vi "Init.vi"(8 "error in (no error)":errorcluster, 9 "C4209 Cfg":T1={"ResourceName"="", "Enable"=FALSE, "Channel"=1, "CalFileName"="", "MeasName"="", "TempDatFile"="", "Power, dBm"=-30.0, "NumPoints"=201, "Start Freq, Hz"=5000000000.0, "Stop Freq, Hz"=6000000000.0, "NumAverages"=20, "Sweep Type"=0} {"Sweep Type" items=["Linear Frequency", "Log Frequency", "Power Sweep", "CW Time"]; "Stop Freq, Hz" format="%_3p"; "Start Freq, Hz" format="%_3p"}, 11 "C4209 PNA":refnum<class "C4209 PNA.lvclass">) -> (0 "error out":errorcluster, 3 "C4209 PNA out":refnum<class "C4209 PNA.lvclass">)   [LabVIEW 2017, in "C4209 PNA.lvclass"]
uses:
  C4209 PNA.lvclass
  N5222A PNA/N5222AConfig.ctl
  C4209 PNA.lvclass/C4209 PNA.ctl
  <instrlib>/CMT S2 Series VNA/CMT S2 Series VNA.lvlib
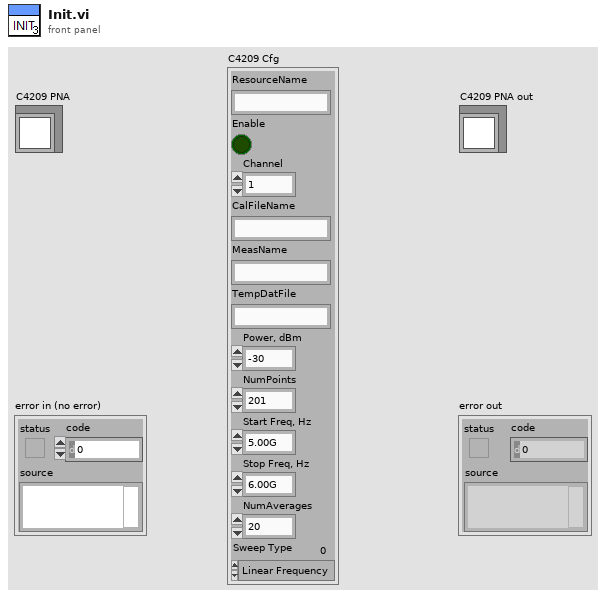
[diagram p1: front panel]
types:
  T1 = typedef "N5222AConfig.ctl" = cluster{"ResourceName":string, "Enable":bool, "Channel":i32, "CalFileName":string, "MeasName":string, "TempDatFile":string, "Power, dBm":dbl, "NumPoints":i32, "Start Freq, Hz":dbl, "Stop Freq, Hz":dbl, "NumAverages":i32, "Sweep Type":i32}
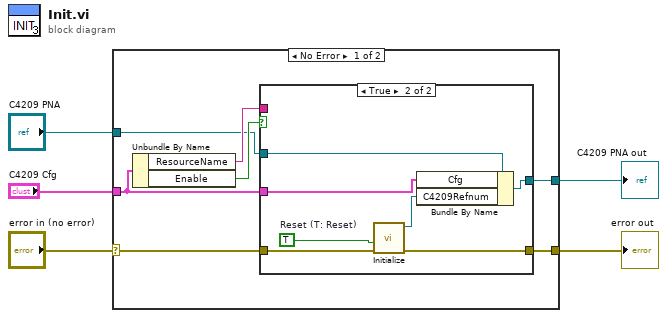
[diagram p0: block diagram]
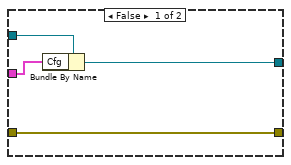
[diagram p2: hidden frame]
diagram:
  n1 = case shown="No Error" "error in (no error)" {
    selector: "error in (no error)" -> [w7 w25]
    tunnel: [w8 w25] -> w4
    tunnel: [w9 w24] -> w2
    tunnel: "C4209 PNA" -> [w10 w24]
    tunnel: "C4209 Cfg" -> [w6 _]
    frame No Error {
      n2 = Unbundle By Name(w6) -> ("ResourceName"=w12:string, "Enable"=w11:bool)
      n3 = case shown="True" w11 {
        tunnel: w12 -> [_ _]
        tunnel: w7 -> [w16 w21]
        tunnel: w10 -> [w14 w23]
        tunnel: [w13 w22] -> w9
        tunnel: w6 -> [w15 w17]
        tunnel: [w16 w19] -> w8
        frame False {
          n4 = Bundle By Name(cluster=w14, "Cfg"=w15) -> (w13:refnum<class "C4209 PNA.lvclass">)
        }
        frame True {
          w20 = TRUE  # Reset (T: Reset)
          n5 = call <instrlib>:"Initialize.vi"("error in (no error)"=w21, "Reset? (T: Yes)"=w20) -> ("error out"=w19:errorcluster, "Reference out"=w18:refnum<k7>)  [unwired: 7 in, 1 out]
          n6 = Bundle By Name(cluster=w23, "Cfg"=w17, "C4209Refnum"=w18) -> (w22:refnum<class "C4209 PNA.lvclass">)
        }
      }
    }
    frame Error {
    }
  }
  "error out" <- w4
  "C4209 PNA out" <- w2
